vi "initializeStyle.vi"(8 "error in (no error)":errorcluster, 10 "Style":refnum<class "Style.lvclass">, 11 "xwpfRun.Figure in":refnum<class "xwpfRun.Figure.lvclass">) -> (0 "error out":errorcluster, 3 "xwpfRun.Figure out":refnum<class "xwpfRun.Figure.lvclass">)   [LabVIEW 2017, in "Word_Specific.lvlib" / "xwpfRun.Figure.lvclass"]
uses:
  xwpfRun.Figure.lvclass
  Styles/Style/Style.lvclass
  Styles/Figure/Figure.lvclass
  C:/Users/Neo/Desktop/Dev_Tools_BR/LabVIEW_NPOI/src/Styles/Style/Style.lvclass
  xwpfRun/xwpfRun.lvclass
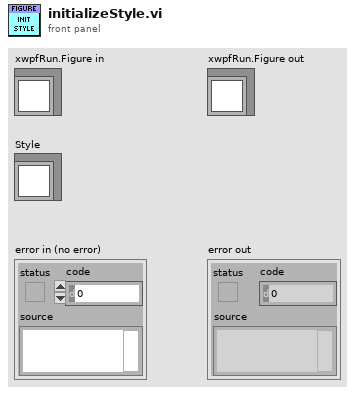
[diagram p1: front panel]
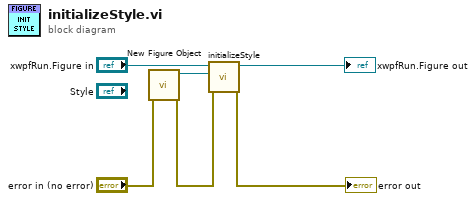
[diagram p0: block diagram]
diagram:
  n1 = call "New Figure Object.vi"("error in (no error)"="error in (no error)") -> ("error out"=w1:errorcluster, "Figure out"=w3:refnum<class "Figure.lvclass">)  [unwired: 9 in]
  n2 = call-parent "initializeStyle.vi"("error in (no error)"=w1, "Style"=w3, "xwpfRun in"="xwpfRun.Figure in") -> ("error out"=→"error out":errorcluster, "xwpfRun out"=→"xwpfRun.Figure out":refnum<class "xwpfRun.Figure.lvclass">)  [unwired: 7 in]
